vi "Set Cell Back Color.vi"(7 "Color":T1, 8 "error in":errorcluster, 9 "Column":i32, 10 "Row":i32, 11 "SourceGrid in":refnum<class "SourceGrid.lvclass">) -> (0 "error out":errorcluster, 3 "SourceGrid out":refnum<class "SourceGrid.lvclass">)   [LabVIEW 2024, in "SourceGrid.lvlib" / "SourceGrid.lvclass"]
uses:
  SourceGrid.lvclass
  System.Drawing.Color.ctl
  SourceGrid.lvclass/SourceGrid.ctl
  Color/Color.lvclass/Color.ctl
  D:/git/Sourcegrid-LabVIEW/dll/SourceGrid.dll
  dll/SourceGrid.dll
  Color/Color.lvclass
  SourceGrid.lvlib
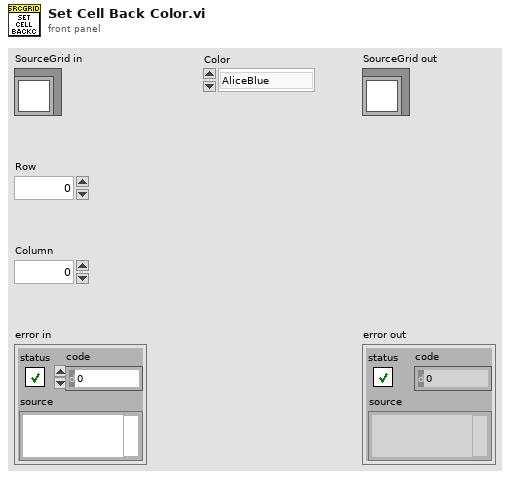
[diagram p1: front panel]
types:
  T1 = typedef "SourceGrid.lvlib/System.Drawing.Color.ctl" = enum16{"AliceBlue", "AntiqueWhite", "Aqua", "Aquamarine", "Azure", "Beige", "Bisque", "Black", "BlanchedAlmond", "Blue", "BlueViolet", "Brown", "BurlyWood", "CadetBlue", "Chartreuse", "Chocolate", "Coral", "CornflowerBlue", "Cornsilk", "Crimson", "Cyan", "DarkBlue", "DarkCyan", "DarkGoldenrod", "DarkGray", "DarkGreen", "DarkKhaki", "DarkMagenta", "DarkOliveGreen", "DarkOrange", "DarkOrchid", "DarkRed", "DarkSalmon", "DarkSeaGreen", "DarkSlateBlue", "DarkSlateGray", "DarkTurquoise", "DarkViolet", "DeepPink", "DeepSkyBlue", "DimGray", "DodgerBlue", "Firebrick", "FloralWhite", "ForestGreen", "Fuchsia", "Gainsboro", "GhostWhite", "Gold", "Goldenrod", "Gray", "Green", "GreenYellow", "Honeydew", "HotPink", "IndianRed", "Indigo", "Ivory", "Khaki", "Lavender", "LavenderBlush", "LawnGreen", "LemonChiffon", "LightBlue", "LightCoral", "LightCyan", "LightGoldenrodYellow", "LightGray", "LightGreen", "LightPink", "LightSalmon", "LightSeaGreen", "LightSkyBlue", "LightSlateGray", "LightSteelBlue", "LightYellow", "Lime", "LimeGreen", "Linen", "Magenta", "Maroon", "MediumAquamarine", "MediumBlue", "MediumOrchid", "MediumPurple", "MediumSeaGreen", "MediumSlateBlue", "MediumSpringGreen", "MediumTurquoise", "MediumVioletRed", "MidnightBlue", "MintCream", "MistyRose", "Moccasin", "NavajoWhite", "Navy", "OldLace", "Olive", "OliveDrab", "Orange", "OrangeRed", "Orchid", "PaleGoldenrod", "PaleGreen", "PaleTurquoise", "PaleVioletRed", "PapayaWhip", "PeachPuff", "Peru", "Pink", "Plum", "PowderBlue", "Purple", "Red", "RosyBrown", "RoyalBlue", "SaddleBrown", "Salmon", "SandyBrown", "SeaGreen", "SeaShell", "Sienna", "Silver", "SkyBlue", "SlateBlue", "SlateGray", "Snow", "SpringGreen", "SteelBlue", "Tan", "Teal", "Thistle", "Tomato", "Transparent", "Turquoise", "Violet", "Wheat", "White", "WhiteSmoke", "Yellow"}
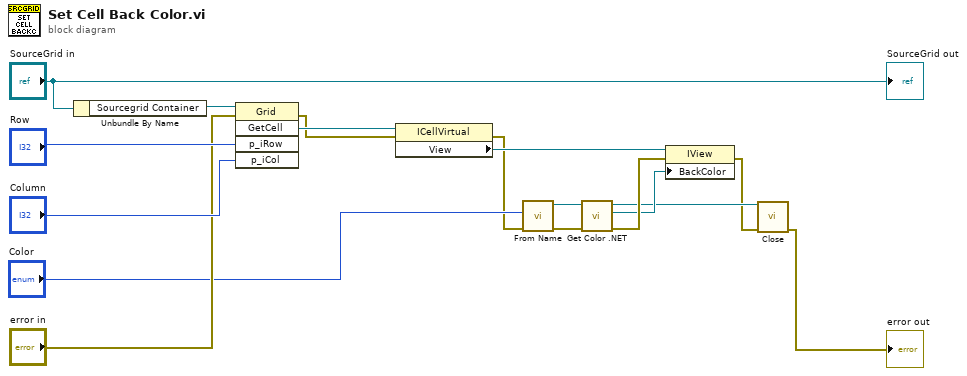
[diagram p0: block diagram]
diagram:
  n1 = Unbundle By Name("SourceGrid in") -> ("Sourcegrid Container"=w15:refnum<k24>)
  n2 = invoke class="Grid" method="GetCell"(reference=w15, error in="error in", "p_iRow"="Row", "p_iCol"="Column") -> (error out=w5:errorcluster, "GetCell"=w6:refnum<k24>)  [unwired: 1 in, 3 out]
  n3 = property class="ICellVirtual"(reference=w6, error in=w5) -> (error out=w8:errorcluster, "View"=w11:refnum<k24>)  [unwired: 1 out]
  n4 = call "From Name.vi"("error in"=w8, "Color"="Color") -> ("error out"=w7:errorcluster, "Color out"=w9:refnum<class "Color.lvclass">)  [unwired: 8 in]
  n5 = call "Get Color .NET.vi"("Color in"=w9) -> ("Color .NET"=w4:refnum<k24>, "Color out"=w3:refnum<class "Color.lvclass">)  [unwired: 9 in]
  n6 = property class="IView"(reference=w11, error in=w7, "BackColor"=w4) -> (error out=w2:errorcluster)  [unwired: 1 out]
  n7 = call-dynamic "Close.vi"("error in"=w2, "Color in"=w3) -> ("error out"=→"error out":errorcluster)  [unwired: 8 in, 1 out]
  "SourceGrid out" <- "SourceGrid in"
